vi "FollowingStepsSubVi.vi"() -> (3 "ArrayOutput":T1)   [LabVIEW 2019]
uses:
  FollowingSteps.ctl
  SpeedAndTimeCluster.ctl
panel:
  in  "ArratDefault":T1
  in  "AcceptProgram":bool
  out "Following Steps":T1
  in  "AddStep":bool
  in  "Speed":u16
  in  "Time":u16
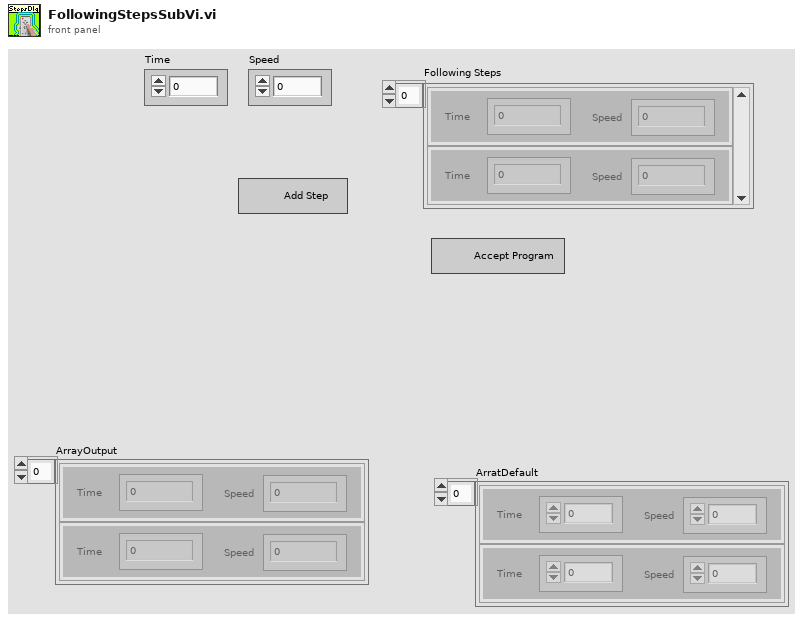
[diagram p1: front panel]
types:
  T1 = typedef "FollowingSteps.ctl" = T2[]
  T2 = typedef "SpeedAndTimeCluster.ctl" = cluster{"Time ":dbl, " Speed":u16}
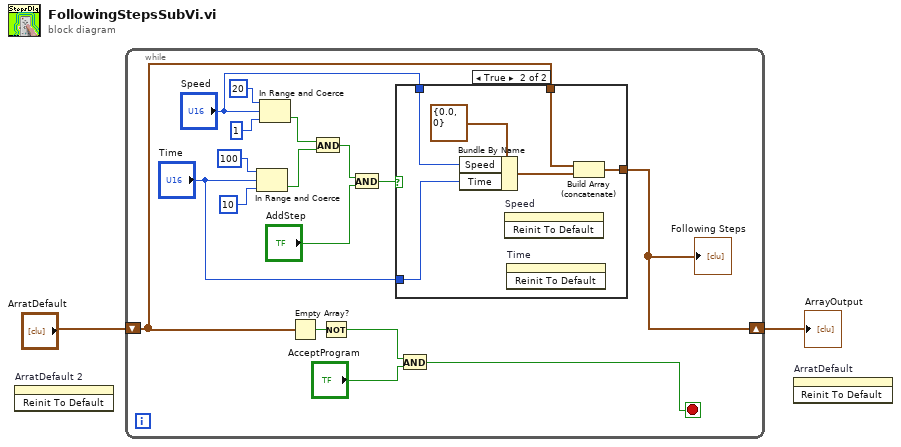
[diagram p0: block diagram]
diagram:
  n1 = invoke on="ArratDefault 2" class="Arr (strict)" method="Reinit To Default"() -> ()  [unwired: 3 in, 3 out]
  n2 = while {
    shift-right: [w5] -> w1
    shift-left: "ArratDefault" -> [w9]
    stop <- w3 stop-if-true
    n3 = In Range and Coerce(upper limit=u16 100, x="Time", lower limit=u16 10) -> (In Range?=w14:bool)  [unwired: 1 out]
    n4 = In Range and Coerce(upper limit=u16 20, x="Speed", lower limit=u16 1) -> (In Range?=w15:bool)  [unwired: 1 out]
    n5 = Empty Array?(array=w9) -> (empty?=w8:bool)
    n6 = And(x=w15, y=w14) -> (x .and. y?=w12:bool)
    n7 = Not(x=w8) -> (.not. x?=w7:bool)
    n8 = And(x=w12, y="AddStep") -> (x .and. y?=w11:bool)
    n9 = case shown="True" w11 {
      tunnel: "Speed" -> [_ w26]
      tunnel: w9 -> [w20 w24]
      tunnel: [w20 w22] -> w5
      tunnel: "Time" -> [_ w21]
      frame False {
      }
      frame True {
        n10 = Bundle By Name(cluster=T2 {"Time "=0.0, " Speed"=0} ("SpeedAndTime"), "Speed"=w26, "Time"=w21) -> (w23:T2)
        n11 = invoke on="Speed" class="DigNum (strict)" method="Reinit To Default"() -> ()  [unwired: 3 in, 3 out]
        n12 = invoke on="Time" class="DigNum (strict)" method="Reinit To Default"() -> ()  [unwired: 3 in, 3 out]
        n13 = Build Array (concatenate)(w24, w23) -> (w22:T1)
      }
    }
    "Following Steps" <- w5
    n14 = And(x=w7, y="AcceptProgram") -> (x .and. y?=w3:bool)
  }
  "ArrayOutput" <- w1
  n15 = invoke on="ArratDefault" class="Arr (strict)" method="Reinit To Default"() -> ()  [unwired: 3 in, 3 out]
